vi "Formula Waveform.vi"(5 "offset":dbl format="%0.2p", 6 "sampling info":cluster{"Fs":dbl, "#s":dbl}={"Fs"=1000.0, "#s"=1000.0} {"Fs" format="%.2p"}, 7 "reset signal":bool, 8 "error in (no error)":errorcluster, 9 "formula":string="sin(w*t)*sin(2*pi(1)*t)", 10 "amplitude":dbl=1.0 format="%0.2p", 11 "frequency":dbl=10.0 format="%0.2p") -> (0 "error out":errorcluster, 3 "signal out":waveform(dbl))   [LabVIEW 2020, in "NI_MAPro.lvlib"]
doc: "Creates an output waveform using a formula string to specify the time function to be used."
uses:
  NI_MAPro.lvlib
  NI_MABase.lvlib
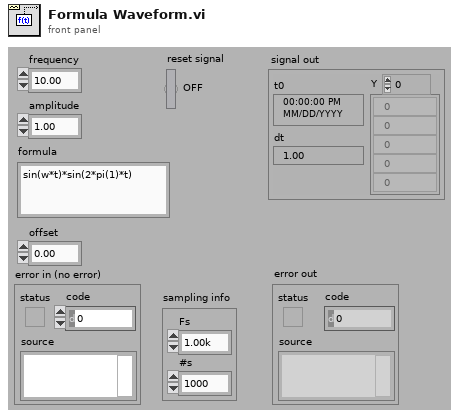
[diagram p1: front panel]
types:
  T1 = cluster{"frequency":dbl, "amplitude":dbl, "formula":string, "sampling info":cluster{"Fs":dbl, "#s":dbl}}
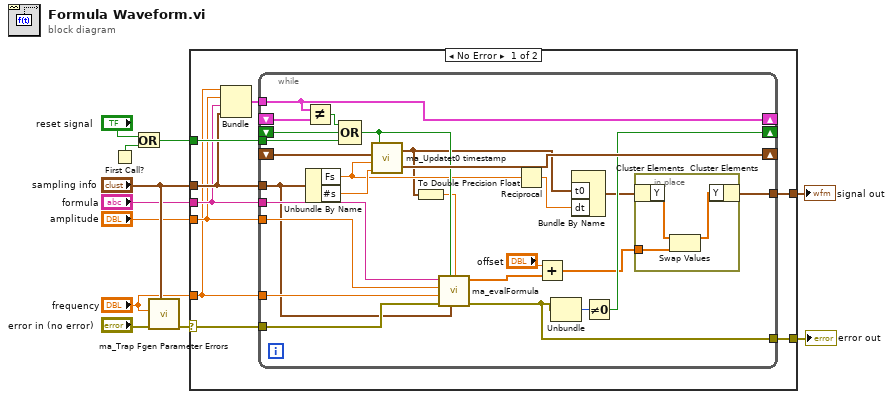
[diagram p0: block diagram]
diagram:
  n1 = First Call?() -> (First Call?: T/F=w9:bool)
  n2 = Or(x="reset signal", y=w9) -> (x .or. y?=w10:bool)
  n3 = call "ma_Trap Fgen Parameter Errors.vi"("Sampling info"="sampling info", "error in (no error)"="error in (no error)", "frequency"="frequency") -> ("error out"=w8:errorcluster)  [unwired: 8 in]
  n4 = case shown="No Error" w8 {
    selector: w8 -> [w18 w51]
    tunnel: w10 -> [w20 _]
    tunnel: "sampling info" -> [w16 _]
    tunnel: "frequency" -> [w13 _]
    tunnel: [w19 w51] -> w5
    tunnel: [w12 _] -> w4
    tunnel: "formula" -> [w15 _]
    tunnel: "amplitude" -> [w14 _]
    frame No Error {
      n5 = Bundle("frequency"=w13, "amplitude"=w14, "formula"=w15, "sampling info"=w16) -> (w17:T1)  [unwired: 1 in]
      n6 = while {
        tunnel: w17 -> [w34]
        shift-left: _ -> [w35]
        shift-right: [w34] -> _
        tunnel: w14 -> [w38]
        tunnel: w18 -> [w40]
        tunnel: w15 -> [w37]
        tunnel: [w28] -> w19
        tunnel: w13 -> [w39]
        tunnel: w16 -> [w36]
        tunnel: w20 -> [w25]
        shift-left: _ -> [w47]
        shift-right: [w46] -> _
        shift-right: [w26] -> _
        shift-left: _ -> [w24]
        tunnel: [w21] -> w12
        stop <- TRUE stop-if-true
        n7 = Not Equal?(x=w34, y=w35) -> (x != y?=w33:bool)
        n8 = Unbundle By Name(w36) -> ("Fs"=w31:dbl, "#s"=w42:dbl)
        n9 = Compound Arithmetic op=OR(w33, w24, w25) -> (w32:bool)
        n10 = call "ma_Updatet0 timestamp.vi"("samples"=w42, "sampling rate (S/s)"=w31, "tf previous"=w47, "Reset Generation"=w32) -> ("tf new"=w46:timestamp, "t0"=w29:timestamp)
        n11 = To Double Precision Float(number=w29) -> (double precision float=w30:dbl)
        n12 = call "ma_evalFormula.vi"("t0"=w30, "Sampling info"=w36, "Reset"=w32, "error in (no error)"=w40, "Frequency"=w39, "Amplitude"=w38, "Formula"=w37) -> ("error out"=w28:errorcluster, "Arbitrary Wave"=w41:dbl[])  [unwired: 3 in]
        n13 = Reciprocal(x=w31) -> (1/x=w44:dbl)
        n14 = Add(x="offset", y=w41) -> (x+y=w23:dbl[])
        n15 = Unbundle(w28) -> ("code"=w27:i32)  [unwired: 2 out]
        n16 = Bundle By Name("t0"=w29, "dt"=w44) -> (w22:waveform(dbl))  [unwired: 1 in]
        n17 = Not Equal To 0?(x=w27) -> (x != 0?=w26:bool)
        n18 = in-place {
          in-place-border: w23 -> [w48]
          n19 = in-place-cluster #1(w22) -> ("Y"=w50:dbl[])
          n20 = Swap Values(12:w50, 14:w48) -> (1:w49:dbl[])  [unwired: 1 in, 1 out]
          n21 = in-place-cluster #1("Y"=w49) -> (w21:waveform(dbl))
        }
      }
    }
    frame Error {
    }
  }
  "error out" <- w5
  "signal out" <- w4
